vi "waitToStopGetClientStatus.vi"(8 "error in (no error)":errorcluster, 11 "tcpServer in":refnum<class "TcpServer.lvclass">) -> (0 "error out":errorcluster, 2 "stop":bool, 3 "tcpServer out":refnum<class "TcpServer.lvclass">)   [LabVIEW 2018, in "TcpServer.lvclass"]
doc: "Wait to stop the getClientStatus.vi. This is a non-block call function."
uses:
  TcpServer.lvclass
  TcpServer.lvclass/TcpServer.ctl
  TcpServerBase/TcpServerBase.lvclass/TcpServerBase.ctl
  TcpServerCmd/TcpServerCmd.lvclass
  home/pcortes/Documents/github/ts_labview_tcp_json/src/TcpServerBase/TcpServerBase.lvclass
  TcpServerBase/TcpServerBase.lvclass
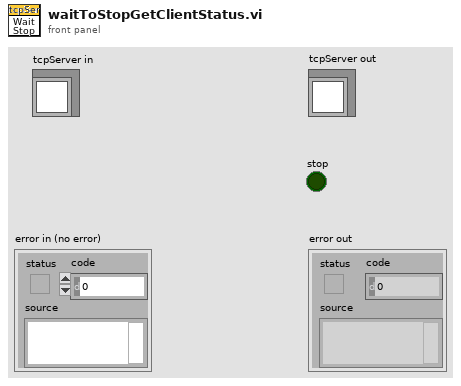
[diagram p1: front panel]
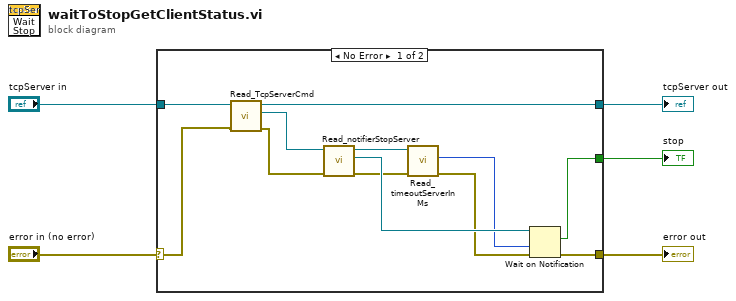
[diagram p0: block diagram]
diagram:
  n1 = case shown="No Error" "error in (no error)" {
    selector: "error in (no error)" -> [w11 w19]
    tunnel: [w14 w19] -> w4
    tunnel: "tcpServer in" -> [w12 w18]
    tunnel: [w13 w18] -> w2
    tunnel: [w15 _] -> w1
    frame No Error {
      n2 = call "Read_TcpServerCmd.vi"("error in (no error)"=w11, "TcpServer in"=w12) -> ("error out"=w16:errorcluster, "TcpServerCmd.lvclass"=w17:refnum<class "TcpServerCmd.lvclass">, "TcpServer out"=w13:refnum<class "TcpServer.lvclass">)  [unwired: 7 in]
      n3 = call "Read_notifierStopServer.vi"("error in (no error)"=w16, "TcpServerBase in"=w17) -> ("error out"=w8:errorcluster, "notifierStopServer"=w10:refnum<notifier>, "TcpServerBase out"=w9:refnum<class "TcpServerCmd.lvclass">)  [unwired: 7 in]
      n4 = call "Read_timeoutServerInMs.vi"("error in (no error)"=w8, "TcpServerBase in"=w9) -> ("error out"=w7:errorcluster, "timeoutServerInMs"=w6:i32)  [unwired: 7 in, 1 out]
      n5 = Wait on Notification(notifier=w10, timeout in ms (-1)=w6, error in (no error)=w7) -> (notification=w15:bool, error out=w14:errorcluster)  [unwired: 1 in, 2 out]
    }
    frame Error {
    }
  }
  "error out" <- w4
  "tcpServer out" <- w2
  "stop" <- w1
